vi "Consumer Loop.vi"(8 "error in (no error)":errorcluster) -> (0 "error out":errorcluster)   [LabVIEW 2013]
doc: "Executes the motion commands."
uses:
  Functional_Global/Typedef_Message_Queue_Action.ctl
  Typedef/Typedef_Motor_Message.ctl
  EMC API/EMC_Typedef_Motor_Parameters.ctl
  Globals/Global Stop.vi
panel:
  out "Iterations":i32
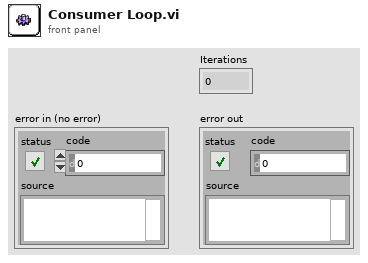
[diagram p1: front panel]
types:
  T1 = typedef "Typedef_Message_Queue_Action.ctl" = enum16{"Init MQueue", "Get MQueue Ref", "Close MQueue"}
  T2 = typedef "Typedef_Motor_Message.ctl" = cluster{"Axis":refnum<k21>, "Motion Parameters":T3}
  T3 = typedef "EMC_Typedef_Motor_Parameters.ctl" = cluster{"position":dbl, "velocity":dbl, "acceleration":dbl, "deceleration":dbl, "accel. jerk":dbl, "decel. jerk":dbl}
  T4 = typedef "Message Queue.lvlib/Message Cluster.ctl" = cluster{"Message":string, "Message Data":variant}
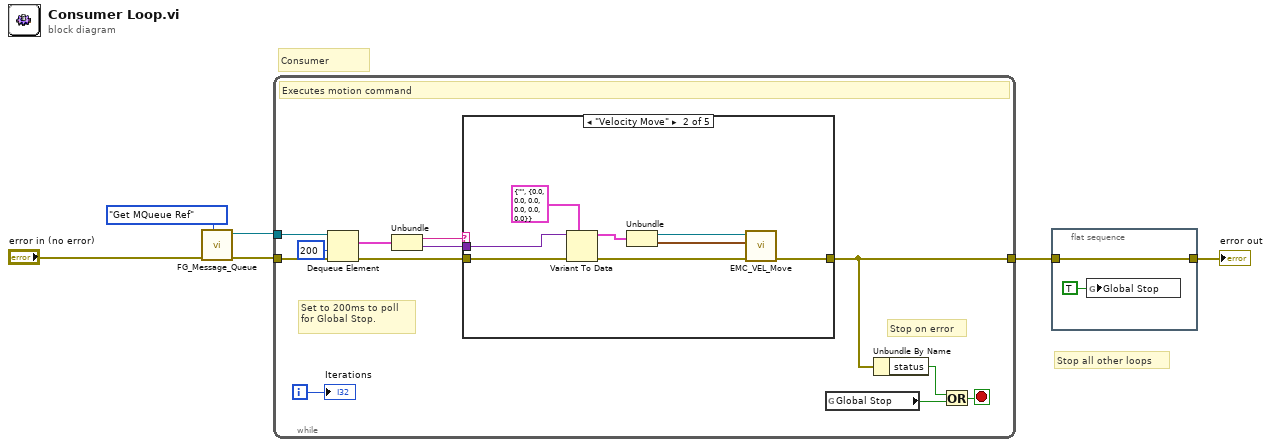
[diagram p0: block diagram]
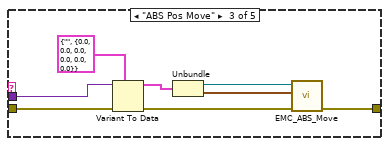
[diagram p3: hidden frame]
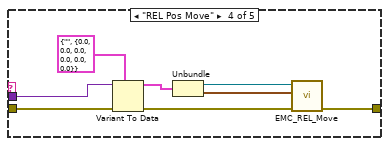
[diagram p4: hidden frame]
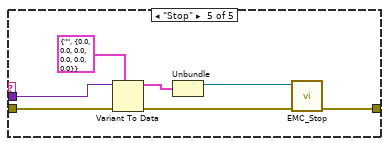
[diagram p5: hidden frame]
diagram:
  # "Stop all other loops"
  # "Consumer"
  n1 = call "FG_Message_Queue.vi"("Action"=Typedef_Message_Queue_Action."Get MQueue Ref", "error in"="error in (no error)") -> ("error out"=w5:errorcluster, "Message Queue"=w4:refnum<queue>)  [unwired: 8 in]
  n2 = while {
    tunnel: w4 -> [w8]
    tunnel: [w11] -> w2
    tunnel: w5 -> [w17]
    i -> [w13]
    stop <- w9 stop-if-true
    # "Stop on error"
    # "Set to 200ms to poll\nfor Global Stop."
    # "Executes motion command"
    n3 = Dequeue Element(queue=w8, timeout in ms (-1)=200, error in (no error)=w17) -> (element=w7:T4, error out=w18:errorcluster)  [unwired: 2 out]
    n4 = Unbundle(w7) -> ("Message"=w16:string, "Message Data"=w15:variant)
    n5 = case shown="\"Velocity Move\"" w16 {
      tunnel: w15 -> [_ w24 w32 w40 w47]
      tunnel: w18 -> [w19 w27 w35 w43 w50]
      tunnel: [w19 w23 w31 w39 w46] -> w11
      frame "Idle", Default {
      }
      frame "Velocity Move" {
        n6 = Variant To Data(error in=w27, type=T2 {"Axis"="", "Motion Parameters"={"position"=0.0, "velocity"=0.0, "acceleration"=0.0, "deceleration"=0.0, "accel. jerk"=0.0, "decel. jerk"=0.0}} ("Motor_Message"), Variant=w24) -> (data=w22:T2, error out=w26:errorcluster)
        n7 = Unbundle(w22) -> ("Axis"=w20:refnum<k21>, "Motion Parameters"=w21:T3)
        n8 = call "EMC_VEL_Move.vi"("error in (no error)"=w26, "Motion Parameters"=w21, "axis"=w20) -> ("error out"=w23:errorcluster)  [unwired: 8 in]
      }
      frame "ABS Pos Move" {
        n9 = Variant To Data(error in=w35, type=T2 {"Axis"="", "Motion Parameters"={"position"=0.0, "velocity"=0.0, "acceleration"=0.0, "deceleration"=0.0, "accel. jerk"=0.0, "decel. jerk"=0.0}} ("Motor_Message"), Variant=w32) -> (data=w30:T2, error out=w34:errorcluster)
        n10 = Unbundle(w30) -> ("Axis"=w28:refnum<k21>, "Motion Parameters"=w29:T3)
        n11 = call "EMC_ABS_Move.vi"("error in (no error)"=w34, "Motion Parameters"=w29, "axis"=w28) -> ("error out"=w31:errorcluster)  [unwired: 8 in]
      }
      frame "REL Pos Move" {
        n12 = Variant To Data(error in=w43, type=T2 {"Axis"="", "Motion Parameters"={"position"=0.0, "velocity"=0.0, "acceleration"=0.0, "deceleration"=0.0, "accel. jerk"=0.0, "decel. jerk"=0.0}} ("Motor_Message"), Variant=w40) -> (data=w38:T2, error out=w42:errorcluster)
        n13 = Unbundle(w38) -> ("Axis"=w36:refnum<k21>, "Motion Parameters"=w37:T3)
        n14 = call "EMC_REL_Move.vi"("error in (no error)"=w42, "Motion Parameters"=w37, "axis"=w36) -> ("error out"=w39:errorcluster)  [unwired: 8 in]
      }
      frame "Stop" {
        n15 = Variant To Data(error in=w50, type=T2 {"Axis"="", "Motion Parameters"={"position"=0.0, "velocity"=0.0, "acceleration"=0.0, "deceleration"=0.0, "accel. jerk"=0.0, "decel. jerk"=0.0}} ("Motor_Message"), Variant=w47) -> (data=w45:T2, error out=w49:errorcluster)
        n16 = Unbundle(w45) -> ("Axis"=w44:refnum<k21>)  [unwired: 1 out]
        n17 = call "EMC_Stop.vi"("error in (no error)"=w49, "axis"=w44) -> ("error out"=w46:errorcluster)  [unwired: 8 in, 1 out]
      }
    }
    n18 = global read "Global Stop.vi" "Global Stop"() -> (w12:bool)
    n19 = Unbundle By Name(w11) -> ("status"=w10:bool)
    n20 = Or(x=w10, y=w12) -> (x .or. y?=w9:bool)
    "Iterations" <- w13
  }
  n21 = flat-sequence {
    tunnel: w2 -> [w51]
    tunnel: [w51] -> w1
    frame #0 {
      n22 = global write "Global Stop.vi" "Global Stop"(TRUE ("stop")) -> ()
    }
  }
  "error out" <- w1
